vi "initialise_raps.vi"(8 "error in (no error)":errorcluster, 11 "State":T1(ring)=enum."Minimized") -> (0 "error out":errorcluster, 2 "FPGA VI Reference":T2, 3 "network streaming queues out":T3)   [LabVIEW 2010]
uses:
  network_streaming_queues_cluster.ctl
  FPGAWrapperMH120124FrameScan_PXI7813R/settings_cluster_framescan.ctl
  common_typedefs/channels_cluster.ctl
  fpgaVIsAndControls/gate_cluster.ctl
  common_typedefs/gate_parameters_cluster.ctl
  FPGAWrapperMH120124FrameScan_PXI7813R/configuration_cluster_framescan.ctl
  fpgaVIsAndControls/DDS_board_init_cluster.ctl
  FPGAWrapperMH120124RAPS_PXI7813R/settings_cluster_raps.ctl
  FPGAWrapperMH120124RAPS_PXI7813R/configuration_cluster_raps.ctl
  FPGA_raps_reference.ctl
  fpgaVIsAndControls/inverse_enum.ctl
  command_enum.ctl
  <vilib>/userDefined/High Color/nirio_resource_hc.ctl
  <vilib>/rvi/interface/nirviOpenFPGA/nirviOpenFPGA.xnode
  FPGA Bitfiles/FPGA_RAPS.lvbitx
  <vilib>/rvi/ClientSDK/nirviWhatTheDeviceIsDoing.ctl
  <vilib>/rvi/interface/nirviMethod/nirviMethod.xnode
  <vilib>/rvi/interface/nirviReadWriteControl/nirviReadWriteControl.xnode
  <vilib>/rvi/interface/common/niFpgaNodeNameForErrorReporting.ctl
  <vilib>/rvi/errors/niLvFpgaWhatHappensToTopLevelVI.ctl
  <vilib>/FPGAPlugInAG/PXI-7813R/niLvFpga_Open_PXI-7813R.vi
  <vilib>/rvi/interface/common/dynamic/niFpgaDynamicAddResources.vi
  <vilib>/FPGAPlugInAG/Dynamic/niLvFpga_Reset_Dynamic.vi
  <vilib>/Utility/error.llb/Error Cluster From Error Code.vi
  <vilib>/rvi/errors/niLvFpgaAdjustHostInterfaceError.vi
  NiFpgaLv.dll
panel:
  # "FSK"
  # "Ramped"
  # "FSK"
  # "Chirp Modus"
  # "Unramped"
  # "BPSK"
  # "Single Tone"
  # "FSK"
  # "Ramped"
  # "FSK"
  # "Chirp Modus"
  # "Unramped"
  # "BPSK"
  # "Single Tone"
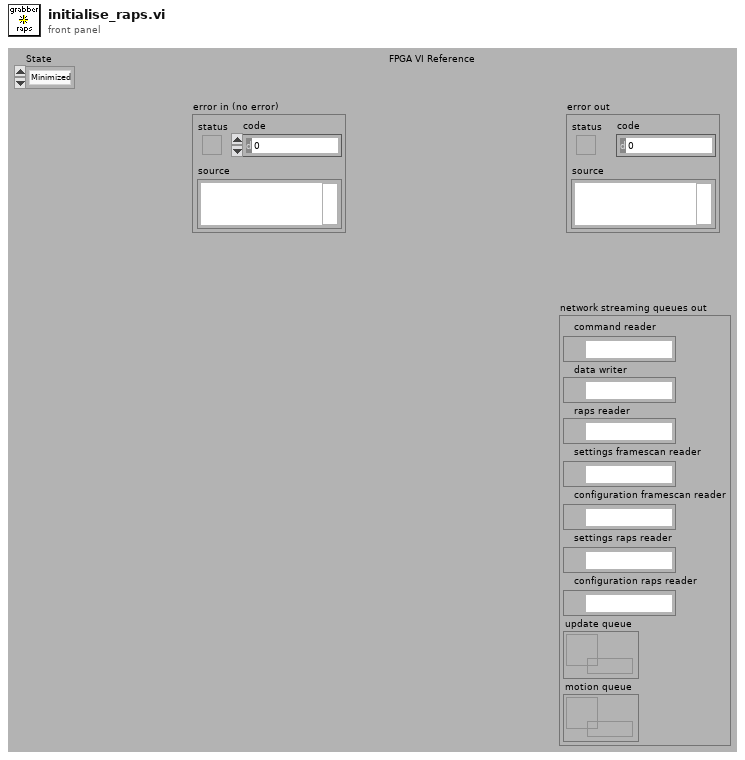
[diagram p1: front panel]
types:
  T1 = enum32{"Invalid", "Standard", "Closed", "Hidden", "Minimized", "Maximized"}
  T2 = typedef "FPGA_raps_reference.ctl" = refnum<k20>
  T3 = typedef "network_streaming_queues_cluster.ctl" = cluster{"command reader":refnum<k21>, "data writer":refnum<k21>, "raps reader":refnum<k21>, "settings framescan reader":refnum<k21>, "configuration framescan reader":refnum<k21>, "settings raps reader":refnum<k21>, "configuration raps reader":refnum<k21>, "update queue":refnum<queue>, "motion queue":refnum<queue>}
  T4 = typedef "inverse_enum.ctl" = enum16{"normal", "x inversed", "y inversed", "x & y inversed"}
  T5 = typedef "command_enum.ctl" = enum8{"NULL", "update", "start", "stop", "reset", "shut-down"}
  T6 = typedef "settings_cluster_raps.ctl" = cluster{"number of pixels":i64, "point package size":u8, "AOD amplitude":u16, "pixel dwell time":dbl, "ra trajectory pixels (data/pixels transfered)":u32, "channel offsets":T7, "offset (Hz)":dbl[], "RAPS array":u64[], "gates":T8[], "enable clocks?":i16, "motion correction":cluster{"# square points":i32, "channel":i8}}
  T7 = typedef "channels_cluster.ctl" = cluster{"channel 0":u32, "channel 1":u32, "channel 2":u32, "channel 3":u32}
  T8 = typedef "gate_cluster.ctl" = cluster{"index":i32, "parameters":T9}
  T9 = typedef "gate_parameters_cluster.ctl" = cluster{"offset":i64, "pulsing":i64, "not pulsing":i64, "cycles per pulse":i64, "repetitions":i64}
  T10 = typedef "configuration_cluster_raps.ctl" = cluster{"DDS board initialization parameters":T11, "OSK select":bool, "AOD equilibration time":dbl, "AOD center frequency":dbl, "AOD Bandwidth":dbl, "inverse?":string, "integration delay (pixels)":u32, "integration delay (iterations)":u32}
  T11 = typedef "DDS_board_init_cluster.ctl" = cluster{"Bypass PLL":bool, "PLL Range":bool, "Update Clock":bool, "Triangle ":bool, "SDO Active":bool, "LSB First":bool, "OSK Int":bool, "Output Shaped Keying Enable":bool, "Bypass Sinc":bool, "Digital Part":bool, "OutPut DAC":bool, "Control DAC":bool, "Comparator":bool, "Modus":u8, "Multiplier Value":u8}
  T12 = typedef "nirio_resource_hc.ctl" = tag
  T13 = typedef "niFpgaNodeNameForErrorReporting.ctl" = enum16{"Open FPGA VI Reference", "Read/Write Control", "Invoke Method: Abort", "Invoke Method: Acknowledge IRQ", "Invoke Method: Download", "Invoke Method: FIFO.Configure", "Invoke Method: FIFO.Read", "Invoke Method: FIFO.Start", "Invoke Method: FIFO.Stop", "Invoke Method: FIFO.Write", "Invoke Method: Reset", "Invoke Method: Run", "Invoke Method: Wait on IRQ", "Close FPGA VI Reference"}
  T14 = typedef "niLvFpgaWhatHappensToTopLevelVI.ctl" = enum16{"top level VI scripted behind XNode", "top level VI inlined behind XNode"}
  T15 = cluster{"AOD Bandwidth_x (Hz)":fxp<+/-,36,32>, "AOD Bandwidth_y (Hz)":fxp<+/-,36,32>, "sin Phi":fxp<+/-,36,2>, "cos Phi":fxp<+/-,36,2>, "Bandwidth for LUTs (256pts)":fxp<+,36,0>, "AOD_Amplitude in":u16, "AOD center frequ. (Hz)_x":fxp<+/-,36,32>, "AOD center frequ. (Hz)_y":fxp<+/-,36,32>, "x offset (Hz)":fxp<+/-,36,32>, "y offset (Hz)":fxp<+/-,36,32>}
  T16 = typedef "nirviWhatTheDeviceIsDoing.ctl" = enum32{"nothing", "something other than LabVIEW FPGA", "FPGA interface", "interactive", "emulation"}
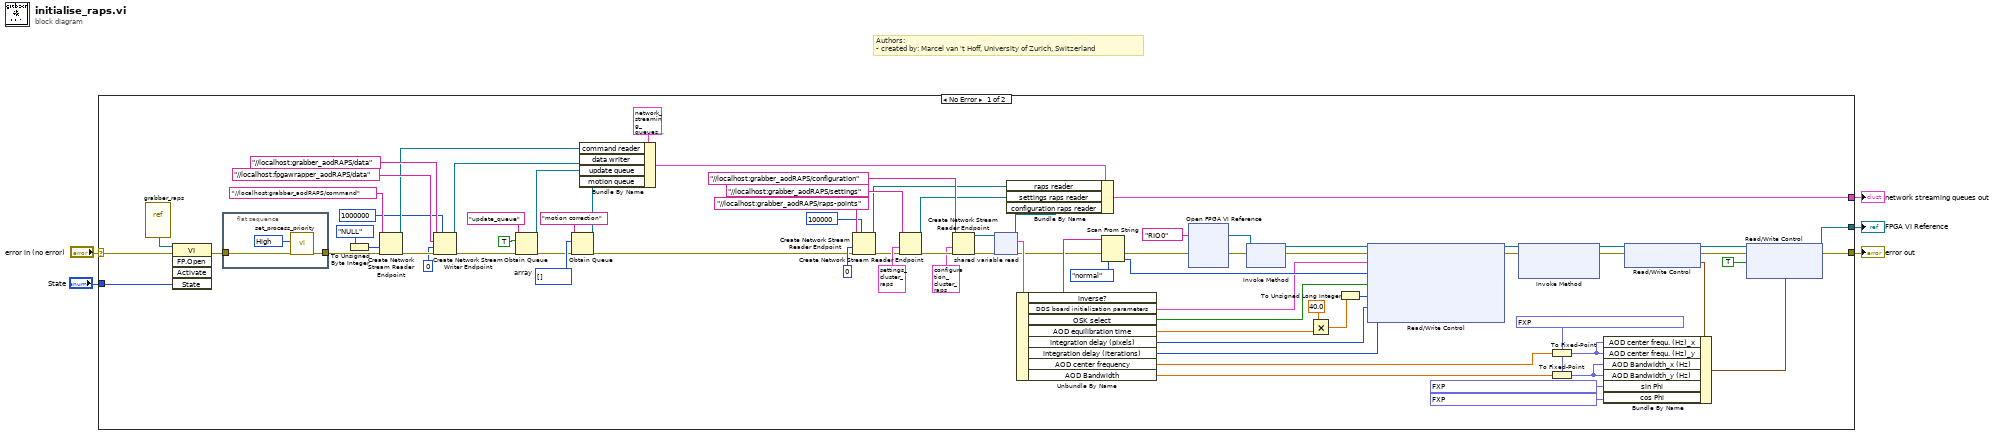
[diagram p0: block diagram]
diagram:
  # "Authors: \n- created by: Marcel van 't Hoff, University of Zurich, Switzerland"
  n1 = case shown="No Error" "error in (no error)" {
    selector: "error in (no error)" -> [w66 w455]
    tunnel: [w70 _] -> w5
    tunnel: [w53 w455] -> w4
    tunnel: [w55 _] -> w2
    tunnel: "State" -> [w6 _]
    frame No Error {
      w10 = u16[] []  # array
      w16 = fxp<+/-,36,32> 0.0 ("sin Phi")
      n2 = vi-ref "grabber_raps.vi"() -> (w67:refnum<vi>)
      n3 = invoke class="VI" method="FP.Open"(reference=w67, error in=w66, "State"=w6) -> (error out=w51:errorcluster)  [unwired: 2 in, 4 out]
      n4 = flat-sequence {
        tunnel: w51 -> [w86]
        tunnel: [w85] -> w36
        frame #0 {
          w84 = 128 items=["Normal"=32, "Idle"=64, "High"=128, "RealTime"=256, "BelowNormal"=16384, "AboveNormal"=32768] ("PriorityClass")
          n5 = call "set_process_priority.vi"("error in (no error)"=w86, "PriorityClass"=w84) -> ("error out"=w85:errorcluster)  [unwired: 9 in]
        }
      }
      n6 = To Unsigned Byte Integer(number=command_enum."NULL" ("command")) -> (unsigned 8bit integer=w47:u8)
      n7 = Create Network Stream Reader Endpoint(8:w36, 9:w47, 11:"//localhost:grabber_aodRAPS/command" ("writer name")) -> (0:w46:errorcluster, 3:w41:refnum<k21>)  [unwired: 3 in]
      n8 = Create Network Stream Writer Endpoint(5:1000000 ("writer buffer size"), 8:w46, 9:u64 0, 10:"//localhost:fpgawrapper_aodRAPS/data" ("reader url"), 11:"//localhost:grabber_aodRAPS/data" ("writer name")) -> (0:w23:errorcluster, 3:w22:refnum<k21>)  [unwired: 1 in]
      n9 = Obtain Queue(name (unnamed)="update_queue", element data type=TRUE, error in (no error)=w23) -> (queue out=w37:refnum<queue>, error out=w9:errorcluster)  [unwired: 2 in, 1 out]
      n10 = Obtain Queue(name (unnamed)="motion correction", element data type=w10, error in (no error)=w9) -> (queue out=w7:refnum<queue>, error out=w8:errorcluster)  [unwired: 2 in, 1 out]
      n11 = Bundle By Name(cluster=T3 {"command reader"="", "data writer"="", "raps reader"="", "settings framescan reader"="", "configuration framescan reader"="", "settings raps reader"="", "configuration raps reader"="", "update queue"=refnum, "motion queue"=refnum} ("network streaming queues"), "command reader"=w41, "data writer"=w22, "update queue"=w37, "motion queue"=w7) -> (w50:T3)
      n12 = Create Network Stream Reader Endpoint(7:100000 ("writer buffer size"), 8:w8, 9:u64 0, 11:"//localhost:grabber_aodRAPS/raps-points" ("reader url")) -> (0:w62:errorcluster, 3:w61:refnum<k21>)  [unwired: 2 in]
      n13 = Create Network Stream Reader Endpoint(8:w62, 9:T6 {"number of pixels"=0, "point package size"=0, "AOD amplitude"=0, "pixel dwell time"=0.0, "ra trajectory pixels (data/pixels transfered)"=0, "channel offsets"={"channel 0"=0, "channel 1"=0, "channel 2"=0, "channel 3"=0}, "offset (Hz)"=[], "RAPS array"=[], "gates"=[], "enable clocks?"=0, "motion correction"={"# square points"=0, "channel"=0}} ("settings cluster"), 11:"//localhost:grabber_aodRAPS/settings" ("reader name")) -> (0:w81:errorcluster, 3:w20:refnum<k21>)  [unwired: 3 in]
      n14 = Create Network Stream Reader Endpoint(8:w81, 9:T10 {"DDS board initialization parameters"={"Bypass PLL"=FALSE, "PLL Range"=FALSE, "Update Clock"=FALSE, "Triangle "=FALSE, "SDO Active"=FALSE, "LSB First"=FALSE, "OSK Int"=FALSE, "Output Shaped Keying Enable"=FALSE, "Bypass Sinc"=FALSE, "Digital Part"=FALSE, "OutPut DAC"=FALSE, "Control DAC"=FALSE, "Comparator"=FALSE, "Modus"=0, "Multiplier Value"=0}, "OSK select"=FALSE, "AOD equilibration time"=0.0, "AOD center frequency"=0.0, "AOD Bandwidth"=0.0, "inverse?"="", "integration delay (pixels)"=0, "integration delay (iterations)"=0} ("configuration cluster"), 11:"//localhost:grabber_aodRAPS/configuration" ("reader name")) -> (0:w80:errorcluster, 3:w79:refnum<k21>)  [unwired: 3 in]
      n15 = shared-variable-read(w79, w80) -> (w21:refnum<k21>, w32:errorcluster, w78:T10)  [unwired: 1 in, 1 out]
      n16 = Bundle By Name(cluster=w50, "raps reader"=w61, "settings raps reader"=w20, "configuration raps reader"=w21) -> (w70:T3)
      n17 = Unbundle By Name(w78) -> ("inverse?"=w34:string, "DDS board initialization parameters"=w19:T11, "OSK select"=w60:bool, "AOD equilibration time"=w29:dbl, "integration delay (pixels)"=w27:u32, "integration delay (iterations)"=w26:u32, "AOD center frequency"=w25:dbl, "AOD Bandwidth"=w24:dbl)
      n18 = Scan From String(input string=w34, error in=w32, default 1=inverse_enum."normal" ("inverse?")) -> (error out=w31:errorcluster, output 1=w30:T4)  [unwired: 2 in, 2 out]
      n19 = xnode "Open FPGA VI Reference"("error in"=w31, "resource name"=T12 "RIO0") -> ("FPGA VI Reference Out"=w83:refnum<k20>, "error out"=w82:errorcluster)
      n20 = xnode "Invoke Method"("FPGA VI Reference In"=w83, "error in"=w82) -> ("FPGA VI Reference Out"=w77:refnum<k20>, "error out"=w76:errorcluster)
      n21 = Multiply(x=40.0, y=w29) -> (x*y=w28:dbl)
      n22 = To Unsigned Long Integer(number=w28) -> (unsigned 32bit integer=w59:u32)
      n23 = xnode "Read/Write Control"("FPGA VI Reference In"=w77, "error in"=w76, "DDS board initialization parameters"=w19, "inverse?"=w30, "OSK select"=w60, "equilibration iterations"=w59, "integration delay (pixels)"=w27, "integration delay (iterations)"=w26) -> ("FPGA VI Reference Out"=w75:refnum<k20>, "error out"=w74:errorcluster)
      n24 = xnode "Invoke Method"("FPGA VI Reference In"=w75, "error in"=w74) -> ("FPGA VI Reference Out"=w52:refnum<k20>, "error out"=w54:errorcluster)  [unwired: 1 in]
      n25 = To Fixed-Point(fixed-point type=w16, number=w25) -> (fixed-point=w17:fxp<+/-,36,32>)
      n26 = To Fixed-Point(fixed-point type=w16, number=w24) -> (fixed-point=w58:fxp<+/-,36,32>)
      n27 = xnode "Read/Write Control"("FPGA VI Reference In"=w52, "error in"=w54) -> ("FPGA VI Reference Out"=w56:refnum<k20>, "error out"=w57:errorcluster, "FPGA parameters"=w13:T15)
      n28 = Bundle By Name(cluster=w13, "AOD center frequ. (Hz)_x"=w17, "AOD center frequ. (Hz)_y"=w17, "AOD Bandwidth_x (Hz)"=w58, "AOD Bandwidth_y (Hz)"=w58, "sin Phi"=fxp<+/-,36,2> 0.0, "cos Phi"=fxp<+/-,36,2> 1.0) -> (w12:T15)
      n29 = xnode "Read/Write Control"("FPGA VI Reference In"=w56, "error in"=w57, "reset in"=TRUE, "FPGA parameters"=w12) -> ("FPGA VI Reference Out"=w55:refnum<k20>, "error out"=w53:errorcluster)
    }
    frame Error {
    }
  }
  "network streaming queues out" <- w5
  "error out" <- w4
  "FPGA VI Reference" <- w2
